vi "Pre-Build Custom Action.vi"(10 "Variant":variant) -> (0 "error out":errorcluster)   [LabVIEW 2020]
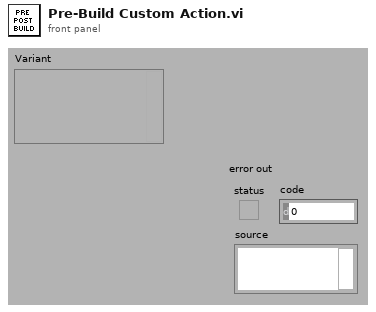
[diagram p1: front panel]
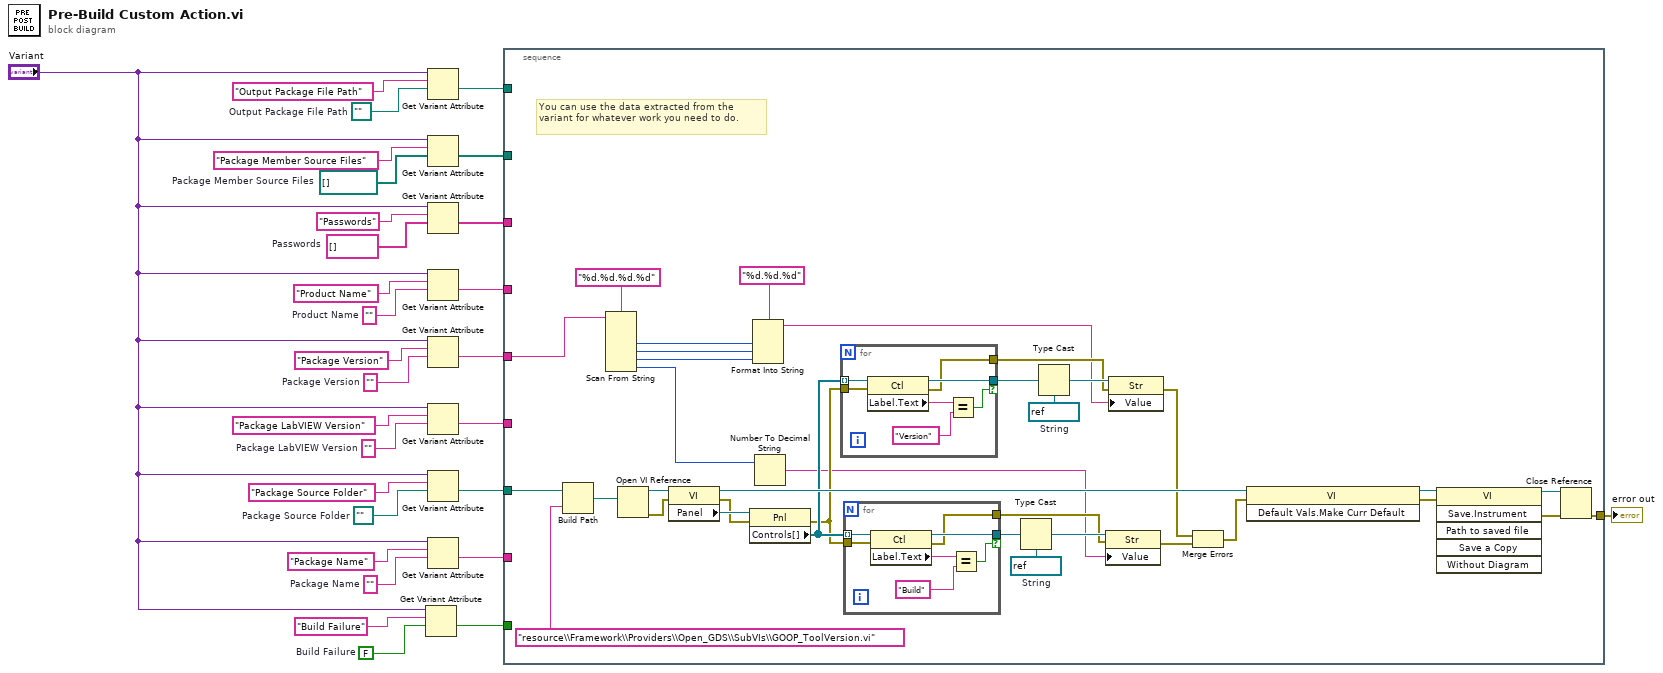
[diagram p0: block diagram]
diagram:
  w4 = FALSE  # Build Failure
  w14 = path ""  # Package Source Folder
  w15 = ""  # Package Name
  w18 = ""  # Package LabVIEW Version
  w20 = ""  # Package Version
  w22 = ""  # Product Name
  w24 = string[] []  # Passwords
  w26 = path[] []  # Package Member Source Files
  w28 = path ""  # Output Package File Path
  n1 = Get Variant Attribute(Variant="Variant", name="Build Failure", default value (empty Variant)=w4) -> (value=w2:bool)  [unwired: 1 in, 3 out]
  n2 = Get Variant Attribute(Variant="Variant", name="Output Package File Path", default value (empty Variant)=w28) -> (value=w13:path)  [unwired: 1 in, 3 out]
  n3 = Get Variant Attribute(Variant="Variant", name="Package Member Source Files", default value (empty Variant)=w26) -> (value=w12:path[])  [unwired: 1 in, 3 out]
  n4 = Get Variant Attribute(Variant="Variant", name="Passwords", default value (empty Variant)=w24) -> (value=w11:string[])  [unwired: 1 in, 3 out]
  n5 = Get Variant Attribute(Variant="Variant", name="Product Name", default value (empty Variant)=w22) -> (value=w10:string)  [unwired: 1 in, 3 out]
  n6 = Get Variant Attribute(Variant="Variant", name="Package Version", default value (empty Variant)=w20) -> (value=w9:string)  [unwired: 1 in, 3 out]
  n7 = Get Variant Attribute(Variant="Variant", name="Package LabVIEW Version", default value (empty Variant)=w18) -> (value=w8:string)  [unwired: 1 in, 3 out]
  n8 = Get Variant Attribute(Variant="Variant", name="Package Source Folder", default value (empty Variant)=w14) -> (value=w7:path)  [unwired: 1 in, 3 out]
  n9 = Get Variant Attribute(Variant="Variant", name="Package Name", default value (empty Variant)=w15) -> (value=w6:string)  [unwired: 1 in, 3 out]
  n10 = stacked-sequence {
    tunnel: w13 -> [_]
    tunnel: w12 -> [_]
    tunnel: w11 -> [_]
    tunnel: w10 -> [_]
    tunnel: w9 -> [w41]
    tunnel: w8 -> [_]
    tunnel: w7 -> [w64]
    tunnel: w6 -> [_]
    tunnel: w2 -> [_]
    tunnel: [w59] -> w1
    frame #0 {
      w38 = refnum<vi> refnum  # String
      w54 = refnum<vi> refnum  # String
      # "You can use the data extracted from the variant for whatever work you need to do."
      n11 = Build Path(base path=w64, name or relative path="resource\\Framework\\Providers\\Open_GDS\\SubVIs\\GOOP_ToolVersion.vi") -> (appended path=w62:path)
      n12 = Scan From String(format string="%d.%d.%d.%d", input string=w41) -> (output 1=w44:i32, output 2=w43:i32, output 3=w42:i32, output 4=w30:i32)  [unwired: 6 in, 3 out]
      n13 = Open VI Reference(vi path=w62) -> (vi reference=w61:refnum<vi>, error out=w57:errorcluster)  [unwired: 5 in]
      n14 = property class="VI"(reference=w61, error in=w57) -> (reference out=w51:refnum<vi>, error out=w58:errorcluster, "Panel"=w60:refnum<vi>)
      n15 = property class="Pnl"(reference=w60, error in=w58) -> (error out=w39:errorcluster, "Controls[]"=w40:refnum<vi>[])  [unwired: 1 out]
      n16 = Format Into String(format string="%d.%d.%d", w44, w43, w42) -> (resulting string=w31:string)  [unwired: 2 in, 1 out]
      n17 = Number To Decimal String(number=w30) -> (decimal integer string=w32:string)  [unwired: 1 in]
      n18 = for {
        tunnel: w40 -> [w71] mode=indexing
        tunnel: [w68] -> w36 if=w67
        tunnel: w39 -> [w66]
        tunnel: [w65] -> w35
        n19 = property class="Ctl"(reference=w71, error in=w66) -> (reference out=w68:refnum<vi>, error out=w65:errorcluster, "Label.Text"=w70:string)
        n20 = Equal?(x=w70, y="Version") -> (x = y?=w67:bool)
      }
      n21 = for {
        tunnel: w40 -> [w78] mode=indexing
        tunnel: [w75] -> w56 if=w74
        tunnel: w39 -> [w73]
        tunnel: [w72] -> w53
        n22 = property class="Ctl"(reference=w78, error in=w73) -> (reference out=w75:refnum<vi>, error out=w72:errorcluster, "Label.Text"=w77:string)
        n23 = Equal?(x=w77, y="Build") -> (x = y?=w74:bool)
      }
      n24 = Type Cast(type=w54, x=w56) -> (*(type *) &x=w55:refnum<vi>)
      n25 = Type Cast(type=w38, x=w36) -> (*(type *) &x=w37:refnum<vi>)
      n26 = property class="Str"(reference=w55, error in=w53, "Value"=w32) -> (error out=w49:errorcluster)  [unwired: 1 out]
      n27 = property class="Str"(reference=w37, error in=w35, "Value"=w31) -> (error out=w33:errorcluster)  [unwired: 1 out]
      n28 = Merge Errors(w33, w49) -> (w34:errorcluster)
      n29 = invoke class="VI" method="Default Vals.Make Curr Default"(reference=w51, error in=w34) -> (reference out=w50:refnum<vi>, error out=w48:errorcluster)  [unwired: 1 in, 1 out]
      n30 = invoke class="VI" method="Save.Instrument"(reference=w50, error in=w48) -> (reference out=w52:refnum<vi>, error out=w47:errorcluster)  [unwired: 4 in, 4 out]
      n31 = Close Reference(reference=w52, error in (no error)=w47) -> (error out=w59:errorcluster)
    }
  }
  "error out" <- w1
